vi "Write Comparison Type.vi"(8 "error in (no error)":errorcluster, 10 "Comparison Type":T1, 11 "Numeric Limit Compare in":refnum<class "Numeric Limit Compare.lvclass">) -> (0 "error out":errorcluster, 3 "Numeric Limit Compare out":refnum<class "Numeric Limit Compare.lvclass">)   [LabVIEW 2015, in "Numeric Limit Compare.lvclass"]
uses:
  Numeric Limit Compare.lvclass
  Config/Comparison Types.ctl
  Numeric Limit Compare.lvclass/Numeric Limit Compare.ctl
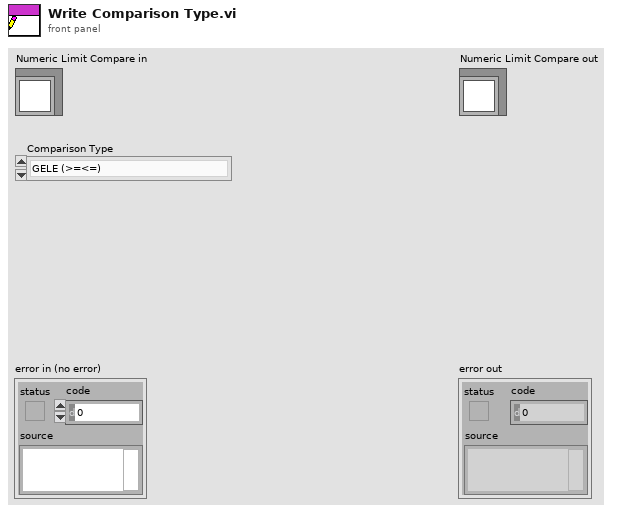
[diagram p1: front panel]
types:
  T1 = typedef "Comparison Types.ctl" = enum16{"GELE (>=<=)", "GTLE(><=)", "GTLT(><)", "GELT(>=<)", "EQ(==)", "NE (!=)", "GT(>)", "LT(<)", "GE(>=)", "LE(<=)"}
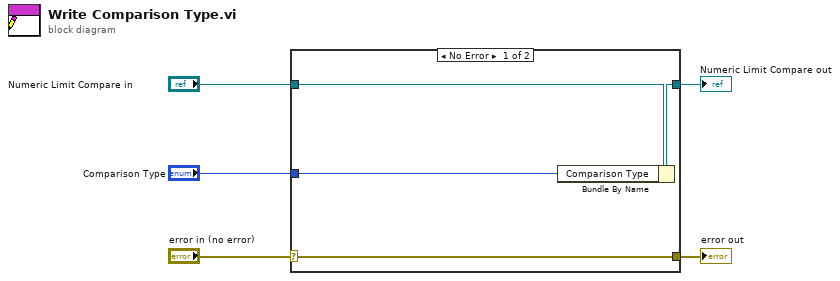
[diagram p0: block diagram]
diagram:
  n1 = case shown="No Error" "error in (no error)" {
    selector: "error in (no error)" -> [w9 w10]
    tunnel: [w9 w10] -> w4
    tunnel: [w7 w11] -> w2
    tunnel: "Numeric Limit Compare in" -> [w8 w11]
    tunnel: "Comparison Type" -> [w6 _]
    frame No Error {
      n2 = Bundle By Name(cluster=w8, "Comparison Type"=w6) -> (w7:refnum<class "Numeric Limit Compare.lvclass">)
    }
    frame Error {
    }
  }
  "error out" <- w4
  "Numeric Limit Compare out" <- w2
